vi "calc_plot_to_smith.vi"(11 "Plot_Data":cluster{"freq_array":dbl[], "X2":dbl[]}[](array[cluster])) -> (3 "smith plot":cluster{"r":dbl, "x":dbl}[](array[cluster])=[{"r"=2.0, "x"=2.0}, {"r"=4.0, "x"=-2.0}])   [LabVIEW 2025]
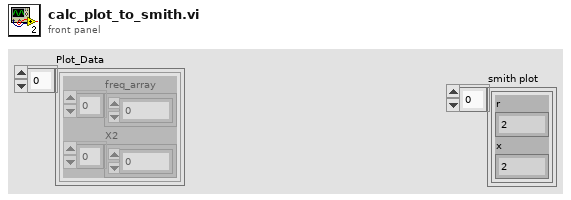
[diagram p1: front panel]
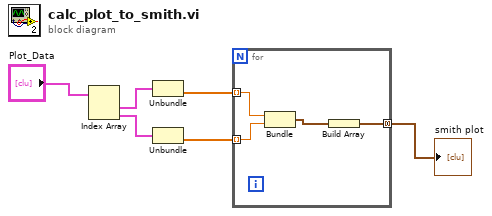
[diagram p0: block diagram]
diagram:
  n1 = Index Array(array="Plot_Data") -> (element #1=w5:cluster{"freq_array":dbl[], "X2":dbl[]}, element #2=w4:cluster{"freq_array":dbl[], "X2":dbl[]})  [unwired: 2 in]
  n2 = Unbundle(w5) -> ("X2"=w3:dbl[])  [unwired: 1 out]
  n3 = Unbundle(w4) -> ("X2"=w2:dbl[])  [unwired: 1 out]
  n4 = for {
    tunnel: [w9] -> w1 mode=concatenating
    tunnel: w3 -> [w8] mode=indexing
    tunnel: w2 -> [w7] mode=indexing
    n5 = Bundle("vswr"=w8, "vswr"=w7) -> (w10:cluster{"vswr":dbl, "vswr":dbl})  [unwired: 1 in]
    n6 = Build Array(w10) -> (w9:cluster{"vswr":dbl, "vswr":dbl}[])
  }
  "smith plot" <- w1
